vi "Database Connection.vi"() -> ()   [LabVIEW 2023]
doc: "This example shows three different methods available to connect to a database: \n\n1) An ODBC data source name (DSN) that has been created from the Control Panel with the Data Sources (ODBC) utility. When you installed the LabVIEW Database Tools, a DSN named LabVIEW was automatically created. This LabVIEW DSN uses the Microsoft Access Driver and refers to the database file labview.mdb in the examples\\database directory.\n\n2) A universal data link (UDL) file created from the LabVIEW Tools>>Create Data Link option. When you installed the LabVIEW Database Tools, the LabVIEW.udl file in the examples\\database directory and UDL file extensions were registered in the Windows registry. \n\n3) A dialog prompt can be used to select the data link properties for a database connection."
uses:
  <vilib>/addons/database/Connection.llb/DB Tools Open Connec (String).vi
  <vilib>/addons/database/Connection.llb/DB Tools Open Connec (Path).vi
  <vilib>/addons/database/NI_Database_API.lvlib
panel:
  out "Connection Succeeded?":bool
  in  "Connection Method":u16(ring) items=["ODBC System DSN", "UDL File", "Prompt"]
  # "Overview: Demonstrates multiple ways to open a connection to a database with the DB Tools Open Connection VI.\nRequirements: Database Connectivity Toolkit\nInstructions:\n1. Select a Connection Method to connect to a database.\n2. Run the VI.\n3. Select a different connection method and run the VI again."
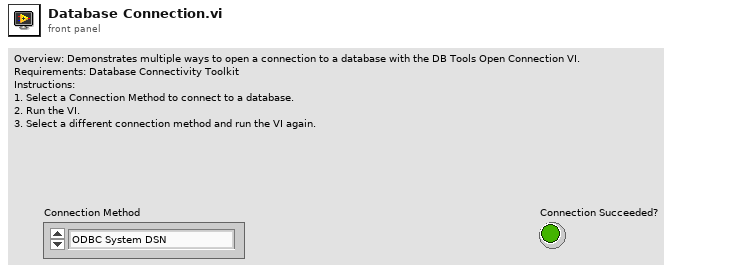
[diagram p1: front panel]
types:
  T1 = typedef "NI_Database_API.lvlib/Conn ObjectReference.ctl" = refnum<k1>
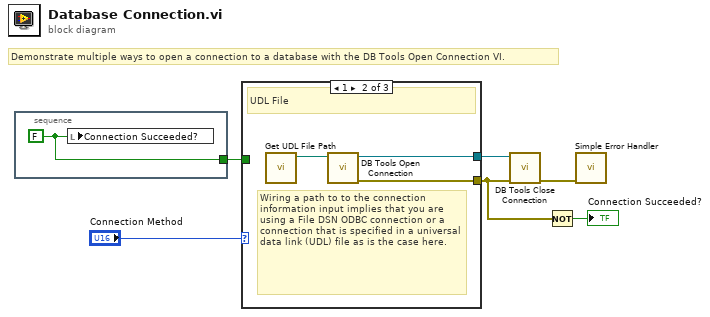
[diagram p0: block diagram]
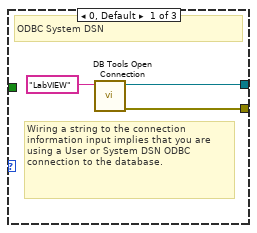
[diagram p2: hidden frame]
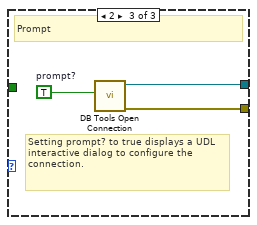
[diagram p3: hidden frame]
diagram:
  # "Demonstrate multiple ways to open a connection to a database with the DB Tools Open Connection VI."
  n1 = stacked-sequence {
    tunnel: [w7] -> w5
    frame #0 {
      w7 = FALSE ("connection succeeded?")
      n2 = local write "Connection Succeeded?"(w7) -> ()
    }
  }
  n3 = case shown="1" "Connection Method" {
    tunnel: [w9 w12 w16] -> w3
    tunnel: [w8 w13 w15] -> w1
    tunnel: w5 -> [_ _ _]
    frame 0, Default {
      # "Wiring a string to the connection information input implies that you are using a User or System DSN ODBC connection to the database."
      # "ODBC System DSN"
      n4 = call-poly <vilib>:"DB Tools Open Connection.vi"("connection information"="LabVIEW") -> ("error out"=w8:errorcluster, "connection reference"=w9:T1)  [unwired: 7 in]
    }
    frame 1 {
      # "Wiring a path to to the connection information input implies that you are using a File DSN ODBC connection or a connection that is specified in a universal data link (UDL) file as is the case here."
      # "UDL File"
      n5 = call "Get UDL File Path.vi"() -> ("UDL file path"=w11:path)  [unwired: 11 in]
      n6 = call-poly <vilib>:"DB Tools Open Connection.vi"("connection information"=w11) -> ("error out"=w13:errorcluster, "connection reference"=w12:T1)  [unwired: 7 in]
    }
    frame 2 {
      w14 = TRUE  # prompt?
      # "Setting prompt? to true displays a UDL interactive dialog to configure the connection."
      # "Prompt"
      n7 = call-poly <vilib>:"DB Tools Open Connection.vi"("prompt? (F)"=w14) -> ("error out"=w15:errorcluster, "connection reference"=w16:T1)  [unwired: 7 in]
    }
  }
  n8 = call <vilib>:"DB Tools Close Connection.vi"("error in (no error)"=w1, "connection reference"=w3) -> ("error out"=w4:errorcluster)  [unwired: 5 in]
  n9 = Not(x=w1) -> (.not. x?=→"Connection Succeeded?":bool)
  n10 = call <vilib>:"Simple Error Handler.vi"("error in (no error)"=w4) -> ()  [unwired: 4 in, 5 out]
